vi "Robot Main.vi"   [LabVIEW 2011]
doc: "This VI imlements the framework and scheduler for your robotics program. It should not be necessary to modify the framework. You are expected to add your code to the VIs called from Robot Main, the ones located in the Team Code within the project."
panel:
  # "ÜberCode 2012!"
  # "questions/comments/complaints can be directed at:\nPhil: http://www.chiefdelphi.com/forums/member.php?u=38911\nJustin: http://www.chiefdelphi.com/forums/member.php?u=39163\n\nOh, and sorry if some of these VIs (like this one) are too big for your\nmonitor. It's what I get for buying a laptop with a 17\" screen"
  # "Version 4.2: Final Code"
  # "What is this code? you might ask. Wonder no more: \nhttp://www.chiefdelphi.com/forums/showpost.php?p=1149162&postcount=8"
  # "Revision History:"
  # "Controls:"
  # "2.2.1:\n-Changed substate typedef and relevent dependencies to use \"auto\" instead of a specific task \n  such as \"shoot\" in order to maintain consistency between loops\n--may need to add separate type defs for loops with multiple\n    functions\n-VI icons\n3.0:\n-turret tuning (still needs more)\n-vision enable FG modifed; uses typedef instead of boolean (added Stop condition)\n-Added competition button mapping\n--fixed state changing\n-auto bridge balancing\n--ability to \"recover\" from tipped bridge\n-added pneumatics loop\n--created new typedef for pneumatic function\n-made code terminate at Finish & closed refnums\n-copeid & modifed WPILib VIs:\n--Joystick get (also outputs an array of \"first press\" buttons\n--Camera MJPEG Loop (added stop condition from vision FG)\n3.2:\n- work on autonomous structure: added proper loop values and such\n- added wait states for pneumatics loop\n- added auto VIs for drive/belts \n- fixed control bugs:\n--turret control: X axis JS3\n--upper belts: Y axis JS2\n--lower belts (^,v): button 3,2 JS2\n- enabled compressor code\n- fixed first call bug with State FG\n- added some static autonomous\n- code is stoppable"
  # "3.3:\n- Added custom dashboard support\n- Added cubic equation for finding desired turret RPS\n- Better turret tracking - changed PID gains, made units consistant, fixed logical errors - turret tracks better\n3.4:\n- Added automatic shooter speed calculation based on target position in image\n-- Battery normalized\n- Additional turret tuning, played with gains\n3.5:\n- Rewrote some aspects of vision/tracking\n-- Static camera settings (exposure/WB -> makes target stand out more in image. wishing for Axis M101)\n-- Tracking rewritten to final revision\n--- Added rational function to determine how much to trust incoming vision values based on drive speed\n---- faster robot is driving, keep more of the newest value. faster correction time, still holds target\n--- added JS3Z Axis to adjust tracking gains\n-- Vision code now has both RGB and HSL filter - finds target better\n3.6:\n- autonomous code added (it's really easy and short with our structure!)\n-- 4 modes: nothing, shoot, get coop bridge then shoot, shoot then coop bridge\n4.0, 4.1:\n- various bits of operational/auto tuning. nothing really new. \n4.2:\n- competition version\n- tweak vision settings for field\n- tweak turret gains for different motor"
  # "Joystick 1:\n- X/Y Axes: Robot Drivetrain (Arcade Drive)\n- Button 1: Hold Drivetrain Position\n- Button 2:  Auto Balancing\n- Button 6:  Shift High\n- Button 7: Raise Bridge Pusher\n- Button 8: Lower Bridge Pusher\n- Button 9: Shift Low\n- Button 10: Retract Extender\n- Button 11: Extender Out\n\nJoystick 2:\n- Y Axis:      Upper Belts\n- Z Axis:      Shooter Speed (Manual Mode)\n- Button 2:  Lower Belts Out\n- Button 3:  Lower Belts In \n- Button 6:  Preset shooter speed, back of key (driver control)\n- Button 7: Preset shooter speed, front of key (driver control)\n- Button 11: raise shooter bias (auto state)\n- Button 10: lower shooter bias (auto state) \n\nJoystick 3:\n- X Axis:           Turret Aim (Manual Mode)\n- Z Axis:           Turret Gains Fine Adjustment\n- Button 1:      Turret to Driver Control\n- Buttons 2-5: Target Selection\n- Button 10:     Reset Turret Encoder\n- Button 11:     Turret Manual Override"
  # "FIRST Team 1124 - The ÜberBots"
  # "http://uberbots.org"
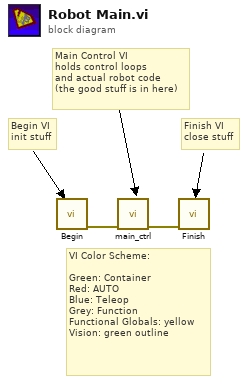
[diagram p0: block diagram]
diagram:
  # "Finish VI\nclose stuff"
  # "Main Control VI\nholds control loops\nand actual robot code\n(the good stuff is in here)"
  # "Begin VI\ninit stuff"
  # "VI Color Scheme:\n\nGreen: Container\nRed: AUTO\nBlue: Teleop\nGrey: Function\nFunctional Globals: yellow\nVision: green outline"
  n1 = call "Begin.vi"() -> ("error out"=w2:errorcluster)  [unwired: 1 in, 10 out]
  n2 = call "main_ctrl.vi"("error in"=w2) -> ("error out"=w1:errorcluster)  [unwired: 10 in]
  n3 = call "Finish.vi"("error in"=w1) -> ()  [unwired: 7 in]
